vi "Licor data processing.vi"(8 "command parameter":T1={"CO2 ref"=392.0, "CO2 span"=372.0, "H2O ref"=0.0, "H2O span"=0.0, "Zi"=0.0, "Zt"=1.2, "Zm"=0.0, "S"=0.0, "Temp [C]"=50.0, "Pressure [hPa]"=135.0, "Licor-Sources"=["CO2A W", "CO2B W", "H2OA W", "H2OB W", "T C", "T V", "P kPa", "P V", "RH %", "CO2A um/m", "CO2B um/m", "H2OA mm/m", "H2OB mm/m"], "Licor-Pump"="Off", "Zeitstempel"=timestamp(0 s since 1904-01-01)} {"Pressure [hPa]" format="%.2g"; "Temp [C]" format="%.2f"; "CO2 ref" format="%.2f"; "CO2 span" format="%.2g"; "H2O ref" format="%.2g"; "H2O span" format="%.2g"}, 9 "mittel CO2B W":dbl[](array[numeric]), 10 "mittel CO2A W":dbl[](array[numeric]), 11 "raw data":string[](array[string])) -> (0 "time; CO2 data":dbl[][](array[numeric]), 1 "mittel CO2B W out":dbl[](array[numeric]), 2 "mittel CO2A W out":dbl[](array[numeric]), 3 "command parameter":T1={"CO2 ref"=0.0, "CO2 span"=0.0, "H2O ref"=0.0, "H2O span"=0.0, "Zi"=0.0, "Zt"=0.0, "Zm"=0.0, "S"=0.0, "Temp [C]"=50.0, "Pressure [hPa]"=135.0, "Licor-Sources"=["CO2A W", "CO2B W", "H2OA W", "H2OB W", "T C", "T V", "P kPa", "P V", "RH %", "CO2A um/m", "CO2B um/m", "H2OA mm/m", "H2OB mm/m"], "Licor-Pump"="Off", "Zeitstempel"=timestamp(0 s since 1904-01-01)} {"Pressure [hPa]" format="%.2g"; "Temp [C]" format="%.2f"; "CO2 ref" format="%.2f"; "CO2 span" format="%.2g"; "H2O ref" format="%.2g"; "H2O span" format="%.2g"})   [LabVIEW 2010]
uses:
  control/Licor-Parameter.ctl
  Licor-Steuerung/LicorLI7000/conventions/Licor-Source.ctl
  control/Licor-Pump.ctl
  Licor-Steuerung/LicorLI7000/LicorLI7000.lvlib
panel:
  out "calibration data out":dbl[][](array[numeric])
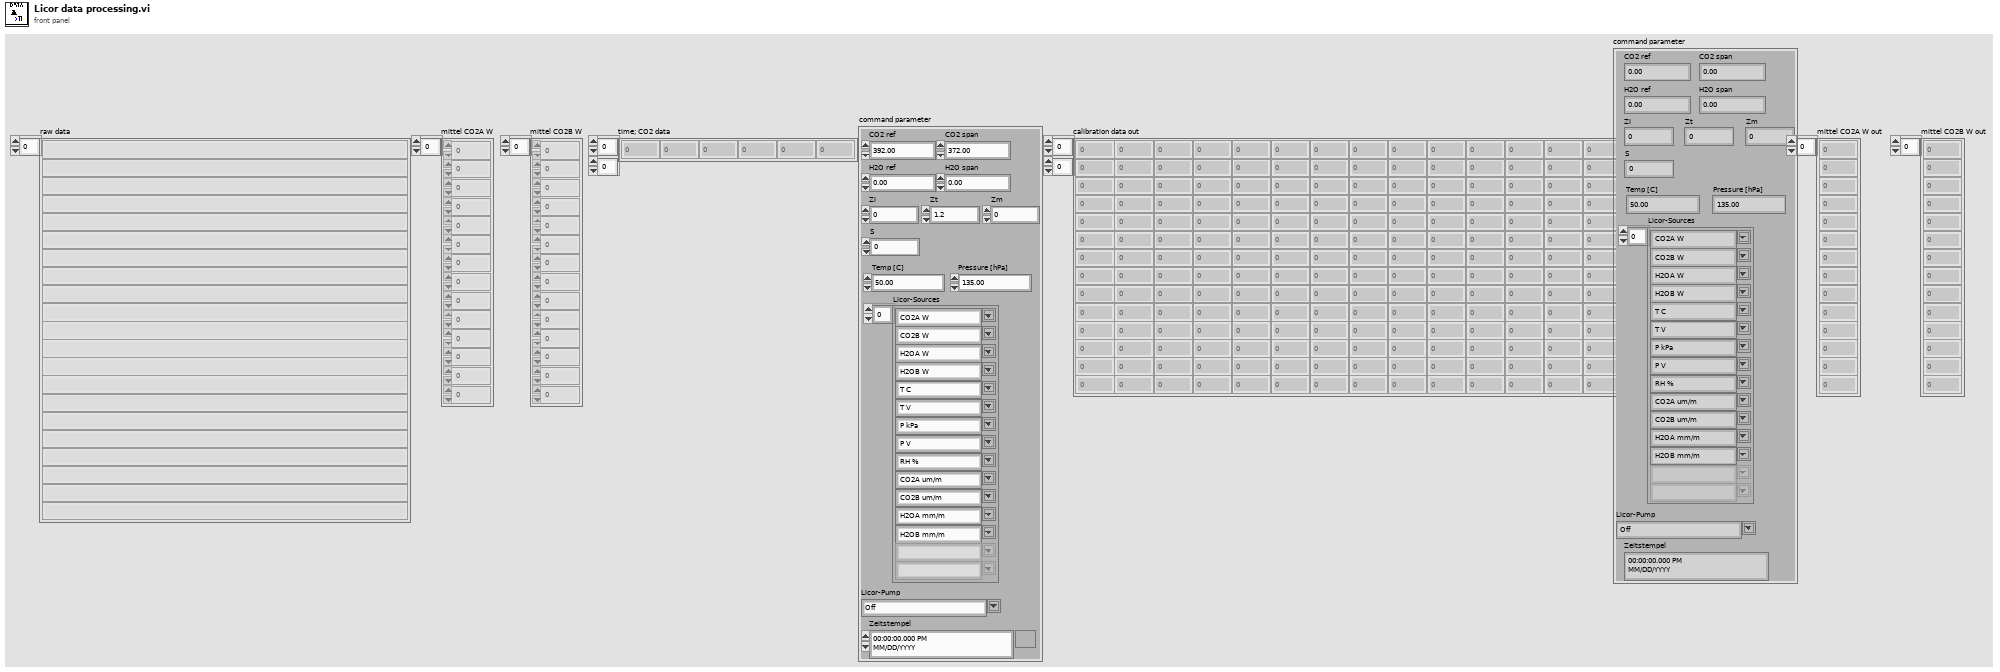
[diagram p1: front panel]
types:
  T1 = typedef "Licor-Parameter.ctl" = cluster{"CO2 ref":dbl, "CO2 span":dbl, "H2O ref":dbl, "H2O span":dbl, "Zi":dbl, "Zt":dbl, "Zm":dbl, "S":dbl, "Temp [C]":dbl, "Pressure [hPa]":dbl, "Licor-Sources":T2[], "Licor-Pump":T3, "Zeitstempel":timestamp}
  T2 = typedef "LicorLI7000.lvlib/Licor-Source.ctl" = string
  T3 = typedef "Licor-Pump.ctl" = string
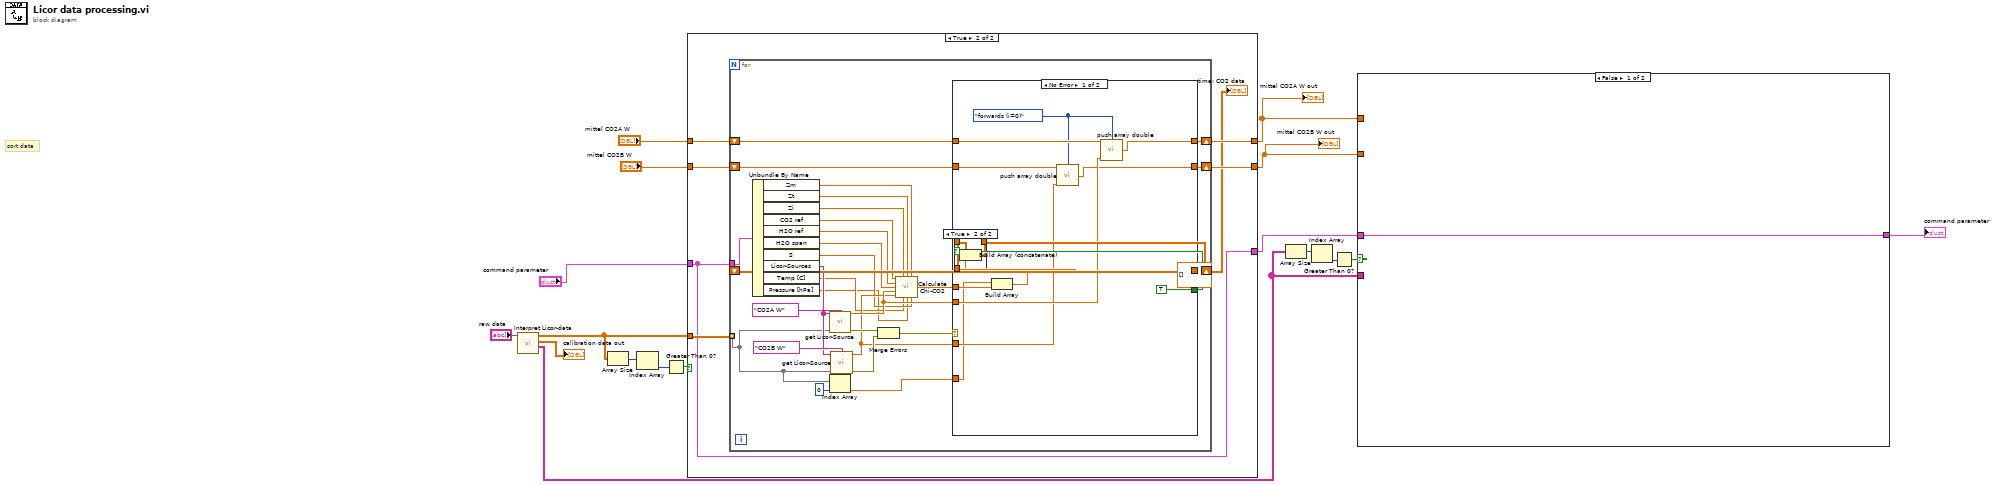
[diagram p0: block diagram]
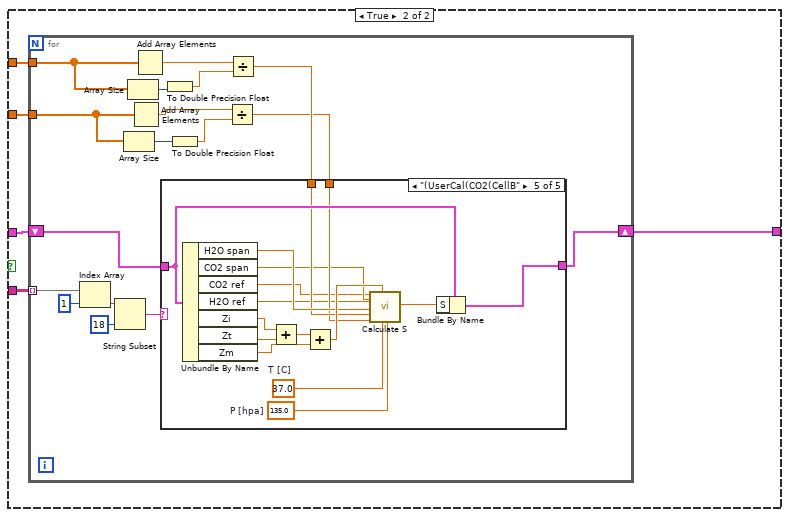
[diagram p2: hidden frame]
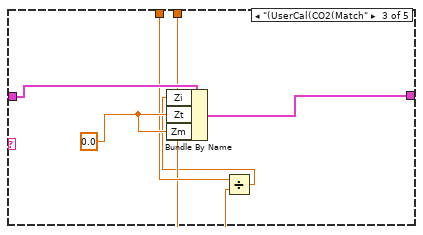
[diagram p5: hidden frame]
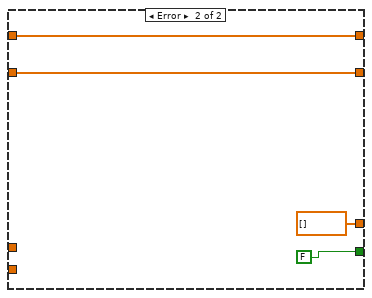
[diagram p9: hidden frame]
diagram:
  # "sort data"
  n1 = call "Interpret Licor-data.vi"("Licor-data"="raw data") -> ("log"=w9:string[][], "calibration data out"=→"calibration data out":dbl[][], "source data out"=w16:dbl[][])  [unwired: 7 in, 1 out]
  n2 = Array Size(array=w16) -> (size(s)=w14:i32[])
  n3 = Index Array(array=w14) -> (element=w13:i32)  [unwired: 1 in]
  n4 = Greater Than 0?(x=w13) -> (x > 0?=w17:bool)
  n5 = case shown="True" w17 {
    tunnel: w16 -> [_ w28]
    tunnel: "command parameter" -> [w20 w27]
    tunnel: [w20 w27] -> w8
    tunnel: "mittel CO2A W" -> [w19 w26]
    tunnel: "mittel CO2B W" -> [w18 w25]
    tunnel: [w19 w24] -> w3
    tunnel: [w18 w23] -> w2
    frame False {
    }
    frame True {
      n6 = for {
        tunnel: w28 -> [w36] mode=indexing
        tunnel: w27 -> [w45]
        shift-right: [w47] -> w24
        shift-left: w26 -> [w49]
        shift-right: [w46] -> w23
        shift-left: w25 -> [w48]
        shift-right: [w29] -> w22
        shift-left: dbl[][] [] ("Array") -> [w30]
        n7 = Unbundle By Name(w45) -> ("Zm"=w53:dbl, "Zt"=w44:dbl, "Zi"=w43:dbl, "CO2 ref"=w42:dbl, "H2O ref"=w41:dbl, "H2O span"=w40:dbl, "S"=w39:dbl, "Licor-Sources"=w38:T2[], "Temp [C]"=w32:dbl, "Pressure [hPa]"=w31:dbl)
        n8 = call "get Licor-Source.vi"("Sources"=w38, "get Source"="CO2A W", "source data"=w36) -> ("value"=w51:dbl, "Fehlerkonstante"=w55:errorcluster)  [unwired: 10 in, 1 out]
        n9 = Index Array(array=w36, index=0 ("Index")) -> (element=w35:dbl)
        n10 = call "get Licor-Source.vi"("Sources"=w38, "get Source"="CO2B W", "source data"=w36) -> ("value"=w50:dbl, "Fehlerkonstante"=w56:errorcluster)  [unwired: 10 in, 1 out]
        n11 = Merge Errors(w55, w56) -> (w54:errorcluster)
        n12 = call "Calculate Chi-CO2.vi"("Chi_CO2_A"=w42, "z_i"=w43, "z_t"=w44, "z_m"=w53, "Chi_H2O_A"=w41, "Chi_H2O_B"=w40, "Raw_CO2_A"=w51, "Raw_CO2_B"=w50, "T [C]"=w32, "P [kPa]"=w31, "S"=w39) -> ("Chi_CO2_B"=w52:dbl)  [unwired: 4 in]
        n13 = case shown="No Error" w54 {
          tunnel: [w64 dbl[] []] -> w34
          tunnel: w52 -> [w73 _]
          tunnel: w50 -> [w66 _]
          tunnel: w51 -> [w71 _]
          tunnel: w49 -> [w72 w77]
          tunnel: w48 -> [w69 w76]
          tunnel: [w70 w77] -> w47
          tunnel: [w67 w76] -> w46
          tunnel: w35 -> [w65 _]
          tunnel: [TRUE FALSE] -> w33
          frame No Error {
            w68 = enum16{"forwards (i=0)", "backwards (i=n)"}."forwards (i=0)" ("mode")
            n14 = Build Array(w65, w73) -> (w64:dbl[])
            n15 = call "push array double.vi"("Array"=w69, "mode"=w68, "Element"=w66) -> ("Array out"=w67:dbl[])  [unwired: 12 in]
            n16 = call "push array double.vi"("Array"=w72, "mode"=w68, "Element"=w71) -> ("Array out"=w70:dbl[])  [unwired: 12 in]
          }
          frame Error {
          }
        }
        n17 = case shown="True" w33 {
          tunnel: w30 -> [w59 w61]
          tunnel: w34 -> [_ w60]
          tunnel: [w59 w62] -> w29
          frame False {
          }
          frame True {
            n18 = Build Array (concatenate)(w61, w60) -> (w62:dbl[][])
          }
        }
      }
      "time; CO2 data" <- w22
    }
  }
  "mittel CO2A W out" <- w3
  "mittel CO2B W out" <- w2
  n19 = Array Size(array=w9) -> (size(s)=w11:i32[])
  n20 = Index Array(array=w11) -> (element=w10:i32)  [unwired: 1 in]
  n21 = Greater Than 0?(x=w10) -> (x > 0?=w7:bool)
  n22 = case shown="False" w7 {
    tunnel: w9 -> [_ w83]
    tunnel: w8 -> [w78 w82]
    tunnel: w2 -> [_ w81]
    tunnel: w3 -> [_ w80]
    tunnel: [w78 w79] -> w1
    frame False {
    }
    frame True {
      n23 = for {
        tunnel: w83 -> [w100] mode=indexing
        shift-right: [w96] -> w79
        shift-left: w82 -> [w84]
        tunnel: w80 -> [w86]
        tunnel: w81 -> [w85]
        n24 = Index Array(array=w100, index=1 ("Index")) -> (element=w97:string)
        n25 = String Subset(string=w97, length (rest)=18 ("Länge (Rest)")) -> (substring=w95:string)  [unwired: 1 in]
        n26 = Array Size(array=w85) -> (size(s)=w93:i32)
        n27 = Array Size(array=w86) -> (size(s)=w92:i32)
        n28 = Add Array Elements(numeric array=w85) -> (sum=w90:dbl)
        n29 = Add Array Elements(numeric array=w86) -> (sum=w94:dbl)
        n30 = To Double Precision Float(number=w92) -> (double precision float=w91:dbl)
        n31 = To Double Precision Float(number=w93) -> (double precision float=w89:dbl)
        n32 = Divide(x=w90, y=w89) -> (x/y=w87:dbl)
        n33 = Divide(x=w94, y=w91) -> (x/y=w88:dbl)
        n34 = case shown="\"(UserCal(CO2(CellB\"" w95 {
          tunnel: w84 -> [w101 w102 w108 w109 w118]
          tunnel: [w101 w102 w107 w109 w119] -> w96
          tunnel: w88 -> [_ _ w105 _ w117]
          tunnel: w87 -> [_ _ w104 _ w116]
          frame "False", Default {
          }
          frame "(UserCal(H2O(Match" {
          }
          frame "(UserCal(CO2(Match" {
            w106 = 0.0 ("Zt")
            n35 = Divide(x=w105, y=w104) -> (x/y=w103:dbl)
            n36 = Bundle By Name(cluster=w108, "Zi"=w103, "Zt"=w106, "Zm"=w106) -> (w107:T1)
          }
          frame "(UserCal(H2O(CellB" {
          }
          frame "(UserCal(CO2(CellB" {
            w123 = 135.0  # P [hpa]
            w122 = 37.0  # T [C]
            n37 = Unbundle By Name(w118) -> ("H2O span"=w121:dbl, "CO2 span"=w115:dbl, "CO2 ref"=w114:dbl, "H2O ref"=w113:dbl, "Zi"=w112:dbl, "Zt"=w111:dbl, "Zm"=w110:dbl)
            n38 = Add(x=w112, y=w111) -> (x+y=w125:dbl)
            n39 = Add(x=w125, y=w110) -> (x+y=w124:dbl)
            n40 = call "Calculate S.vi"("Chi_CO2_A"=w114, "Chi_CO2_B"=w115, "Chi_H2O_A"=w113, "Chi_H2O_B"=w121, "Raw_CO2_A"=w117, "Raw_CO2_B"=w116, "Z"=w124, "T [C]"=w122, "P [hpa]"=w123) -> ("S"=w120:dbl)  [unwired: 10 in]
            n41 = Bundle By Name(cluster=w118, "S"=w120) -> (w119:T1)
          }
        }
      }
    }
  }
  "command parameter" <- w1
